vi "Read Supported Functions.vi"(8 "error in (no error)":errorcluster, 11 "Temperature Controller in":refnum<class "Mag Lab Temperature Controller.lvclass">) -> (0 "error out":errorcluster, 2 "Supported Functions":T1[](array[typedef]), 3 "Temperature Controller out":refnum<class "Mag Lab Temperature Controller.lvclass">)   [LabVIEW 2015, in "Mag Lab Temperature Controller.lvclass"]
uses:
  Mag Lab Temperature Controller.lvclass
  Mag Lab Hardware Function.ctl
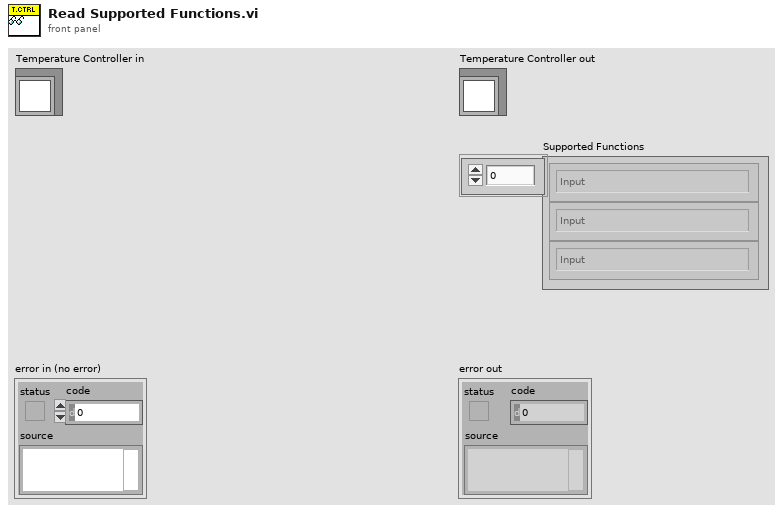
[diagram p1: front panel]
types:
  T1 = typedef "Mag Lab Hardware Function.ctl" = enum16{"Input", "Voltmeter", "Output", "Current source", "Digitizer", "Temperature controller"}
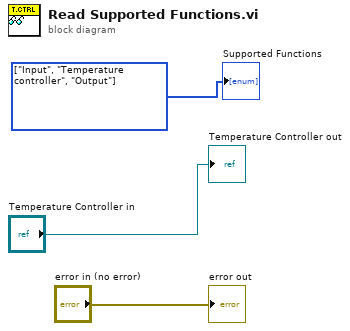
[diagram p0: block diagram]
diagram:
  w1 = T1[] [enum."Input", enum."Temperature controller", enum."Output"] items=["Input", "Voltmeter", "Output", "Current source", "Digitizer", "Temperature controller"] ("Supported Functions")
  "error out" <- "error in (no error)"
  "Temperature Controller out" <- "Temperature Controller in"
  "Supported Functions" <- w1
